vi "AE - Bluetooth LED.vi"(8 "error in (no error)":errorcluster, 10 "LED State":u8, 11 "Wiimote":u8) -> (0 "error out":errorcluster)   [LabVIEW 2010]
uses:
  AE Cores/AE - Bluetooth Enum.ctl
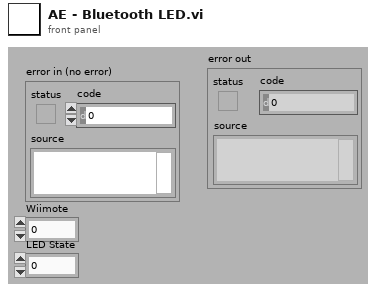
[diagram p1: front panel]
types:
  T1 = typedef "AE - Bluetooth Enum.ctl" = enum16{"Initialise", "Pair All Wiimotes", "Connect All Wiimotes", "Set Rumble", "Set LED", "Get Button + Acc Data", "Get IR Data", "Get Battery", "Get Wiimote Reference", "Reorder Wiimotes", "devReport"}
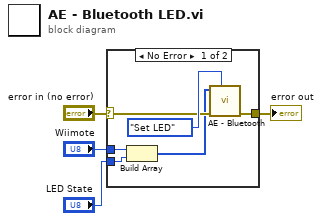
[diagram p0: block diagram]
diagram:
  n1 = case shown="No Error" "error in (no error)" {
    selector: "error in (no error)" -> [w9 w11]
    tunnel: [w8 w11] -> w3
    tunnel: "Wiimote" -> [w7 _]
    tunnel: "LED State" -> [w6 _]
    frame No Error {
      n2 = Build Array(w7, w6) -> (w5:u8[])
      n3 = call "AE - Bluetooth.vi"("Enum"=AE_-_Bluetooth_Enum."Set LED", "error in (no error)"=w9, "Variant In"=w5) -> ("error out"=w8:errorcluster)  [unwired: 6 in, 2 out]
    }
    frame Error {
    }
  }
  "error out" <- w3
